vi "Data_NotchFilter.vi"(6 "Filter Enable":bool, 8 "Notch Filter":u16=60, 11 "Data (Codes)":i32[](array[numeric])) -> (1 "Notch Filter Disable Property":T1=2 items=["Enable", "Disable", "Disable/Gray"], 3 "Filtered Data":i32[](array[numeric]))   [LabVIEW 2010]
doc: "This VI implements a digital notch filter on the input data. The digital filter is a cascade of 2 2nd order IIR notch filters.\nThe input data should be at a data rate = 500SPS.\n\nInputs:\nData (Codes) - (I32[]) data @ 500SPS to be filtered\nNotch Filter - (enum) selection of 50 or 60 Hz notch filter\nFilter Enable - (bool) enable filtering (TRUE=filter, FALSE=pass through)\n\nOutputs:\nFilter Data - (I32[]) data @ 500SPS filtered\nNotch Filter Disable Property - (ring) uses Filter Enable input to set the property for the Notch Filter enum selector"
uses:
  Controls/Misc/TYP_DisableProp.ctl
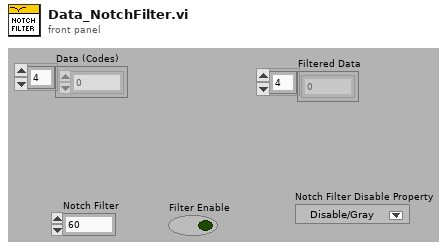
[diagram p1: front panel]
types:
  T1 = typedef "TYP_DisableProp.ctl" = u8
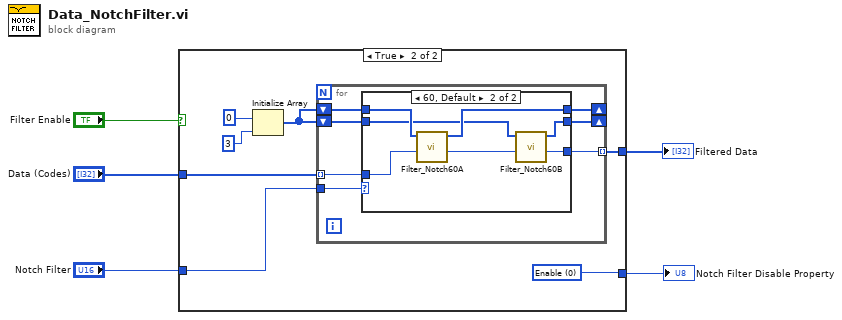
[diagram p0: block diagram]
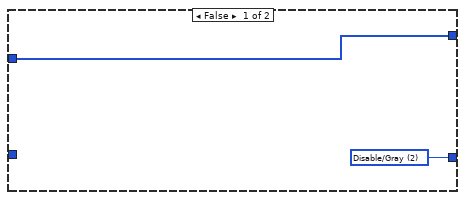
[diagram p2: hidden frame]
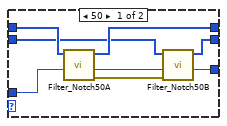
[diagram p3: hidden frame]
diagram:
  n1 = case shown="True" "Filter Enable" {
    tunnel: "Data (Codes)" -> [w6 w11]
    tunnel: [w6 w10] -> w1
    tunnel: [w7 w14] -> w3
    tunnel: "Notch Filter" -> [_ w8]
    frame False {
      w7 = T1 2 items=["Enable", "Disable", "Disable/Gray"] ("Disable Property")
    }
    frame True {
      w14 = T1 0 items=["Enable", "Disable", "Disable/Gray"] ("Disable Property")
      n2 = Initialize Array(0 ("Notch Filter"), 3 ("Notch Filter")) -> (w9:i32[])
      n3 = for {
        tunnel: w11 -> [w21] mode=indexing
        tunnel: [w20] -> w10 mode=indexing
        shift-right: [w19] -> _
        shift-left: w9 -> [w18]
        shift-right: [w17] -> _
        shift-left: w9 -> [w16]
        tunnel: w8 -> [w15]
        n4 = case shown="60, Default" w15 {
          tunnel: w21 -> [w29 w36]
          tunnel: [w27 w34] -> w20
          tunnel: [w26 w33] -> w19
          tunnel: w18 -> [w25 w32]
          tunnel: [w24 w31] -> w17
          tunnel: w16 -> [w23 w30]
          frame 50 {
            n5 = call "Filter_Notch50A.vi"("Input Data"=w29, "Delay Data"=w25) -> ("error out"=w22:errorcluster, "Filtered Data"=w28:i32, "Delay Data out"=w26:i32[])  [unwired: 1 in, 6 out]
            n6 = call "Filter_Notch50B.vi"("error in (no error)"=w22, "Input Data"=w28, "Delay Data"=w23) -> ("Filtered Data"=w27:i32, "Delay Data out"=w24:i32[])  [unwired: 7 out]
          }
          frame 60, Default {
            n7 = call "Filter_Notch60A.vi"("Input Data"=w36, "Delay Data"=w32) -> ("Filtered Data"=w35:i32, "Delay Data out"=w33:i32[])  [unwired: 2 in, 6 out]
            n8 = call "Filter_Notch60B.vi"("Input Data"=w35, "Delay Data"=w30) -> ("Filtered Data"=w34:i32, "Delay Data out"=w31:i32[])  [unwired: 2 in, 6 out]
          }
        }
      }
    }
  }
  "Notch Filter Disable Property" <- w3
  "Filtered Data" <- w1
